vi "Initialize MHL Queue.vi"(3 "error in (no error)":errorcluster) -> (7 "Queue out":refnum<queue>, 10 "error out":errorcluster)   [LabVIEW 2024]
uses:
  Message Cluster.ctl
  Message.ctl
panel:
  in  "Message Cluster":T1={"Message"=enum."UpdateDisplay", "Message Data"=variant(string "")}
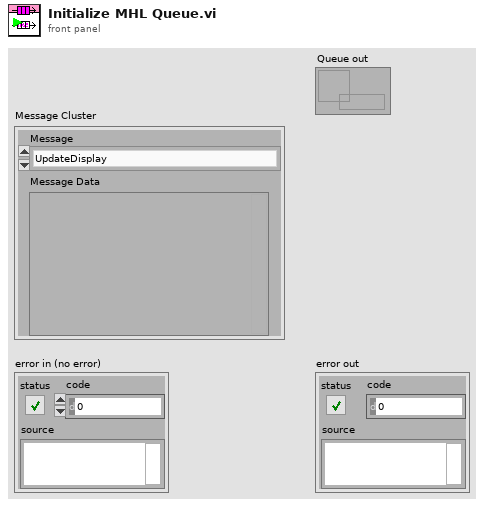
[diagram p1: front panel]
types:
  T1 = typedef "Message Cluster.ctl" = cluster{"Message":T2, "Message Data":variant}
  T2 = typedef "Message.ctl" = enum16{"UpdateDisplay", "Run Washing", "Exit", "Slider run", "Checking wash step", "Continuing washing", "Waiting for slider movement", "Initialize"}
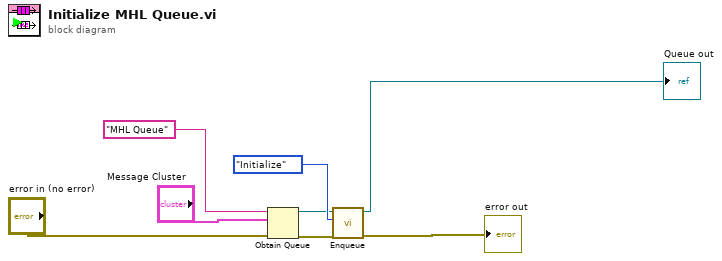
[diagram p0: block diagram]
diagram:
  n1 = Obtain Queue(name (unnamed)="MHL Queue", element data type="Message Cluster", error in (no error)="error in (no error)") -> (queue out=w6:refnum<queue>, error out=w4:errorcluster)  [unwired: 2 in, 1 out]
  n2 = call "Enqueue.vi"("error in (no error)"=w4, "Message"=Message."Initialize", "Message Queue"=w6) -> ("error out"=→"error out":errorcluster, "Message Queue out"=→"Queue out":refnum<queue>)  [unwired: 7 in]
